vi "CheckForCAEN.vi"(10 "error in":errorcluster, 11 "Network Session":refnum<k5>) -> (0 "error out":errorcluster, 1 "Boolean":bool, 2 "String":string, 3 "TCP Network Connection Refnum":refnum<k5>)   [LabVIEW 2025]
doc: "Author: Scott Hannahs <sth@magnet.fsu.edu>\n\nThis software is licensed for use under the “MIT License\"\nCopyright (c) 2025 Scott Hannahs, sth@sth@magnet.sthnet.net\n\nPermission is hereby granted, free of charge, to any person obtaining a copy of this software and associated documentation files (the \"Software\"), to deal in the Software without restriction, including without limitation the rights to use, copy, modify, merge, publish, distribute, sublicense, and/or sell copies of the Software, and to permit persons to whom the Software is furnished to do so, subject to the following conditions: The above copyright notice and this permission notice shall be included in all copies or substantial portions of the Software.\n\nTHE SOFTWARE IS PROVIDED \"AS IS\", WITHOUT WARRANTY OF ANY KIND, EXPRESS OR IMPLIED, INCLUDING BUT NOT LIMITED TO THE WARRANTIES OF MERCHANTABILITY, FITNESS FOR A PARTICULAR PURPOSE AND NONINFRINGEMENT. IN NO EVENT SHALL THE AUTHORS OR COPYRIGHT HOLDERS BE LIABLE FOR ANY CLAIM, DAMAGES OR OTHER LIABILITY, WHETHER IN AN ACTION OF CONTRACT, TORT OR OTHERWISE, ARISING FROM, OUT OF OR IN CONNECTION WITH THE SOFTWARE OR THE USE OR OTHER DEALINGS IN THE SOFTWARE."
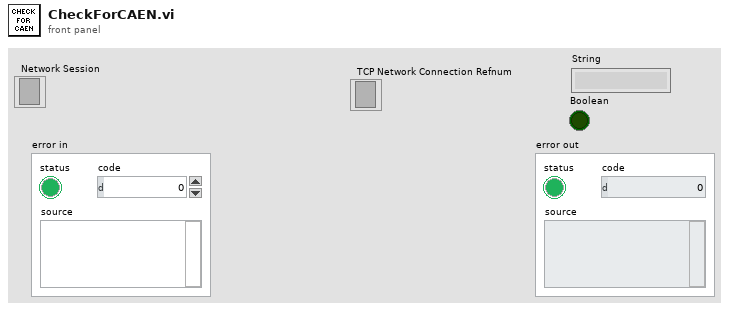
[diagram p1: front panel]
types:
  T1 = enum16{"Standard", "Buffered", "CRLF", "Immediate"}
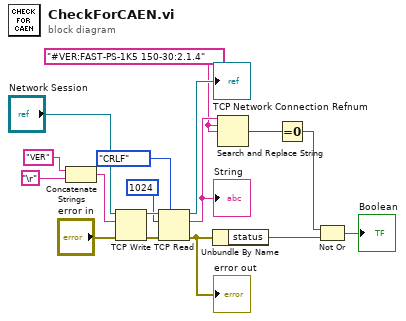
[diagram p0: block diagram]
diagram:
  w4 = "#VER:FAST-PS-1K5 150-30:2.1.4"
  n1 = Concatenate Strings("VER", "\r") -> (w9:string)
  n2 = TCP Write(connection ID="Network Session", data in=w9, error in (no error)="error in") -> (connection ID out=w16:refnum<k5>, error out=w15:errorcluster)  [unwired: 1 in, 1 out]
  n3 = TCP Read(connection ID=w16, bytes to read=1024, error in (no error)=w15, 7:T1."CRLF" ("mode (standard)")) -> (connection ID out=→"TCP Network Connection Refnum":refnum<k5>, data out=w5:string, error out=w12:errorcluster)  [unwired: 1 in]
  "error out" <- w12
  "String" <- w5
  n4 = Unbundle By Name(w12) -> ("status"=w11:bool)
  n5 = Search and Replace String(input string=w5, search string=w4, replace string=w4) -> (number of replacements=w3:i32)  [unwired: 5 in, 3 out]
  n6 = Equal To 0?(x=w3) -> (x = 0?=w2:bool)
  n7 = Not Or(1:w11, 2:w2) -> (0:→"Boolean":bool)
